vi "DVR Example.vi"() -> ()   [LabVIEW 2015]
uses:
  <vilib>/Erdos Miller/LV-VI/Check Out Ref.vi
  <vilib>/Erdos Miller/LV-VI/Check In Ref.vi
  <vilib>/Erdos Miller/LV-Async/async-xnode/LV-Async.xnode
  <vilib>/Erdos Miller/LV-Async/await-xnode/LV-Await.xnode
  <vilib>/Erdos Miller/LV-VI/LV-VI.lvlib
panel:
  out "data value out 2":dbl
  out "error out 2":errorcluster
  out "error out":errorcluster
  out "data value out":dbl
  in  "data value":dbl
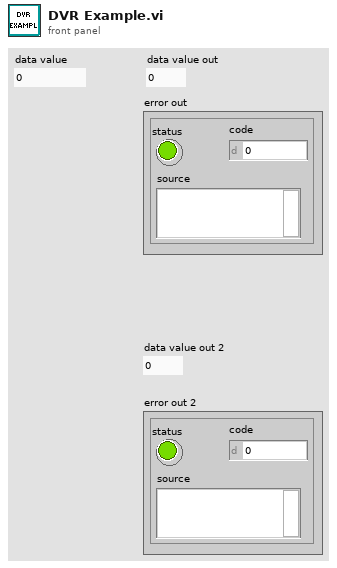
[diagram p1: front panel]
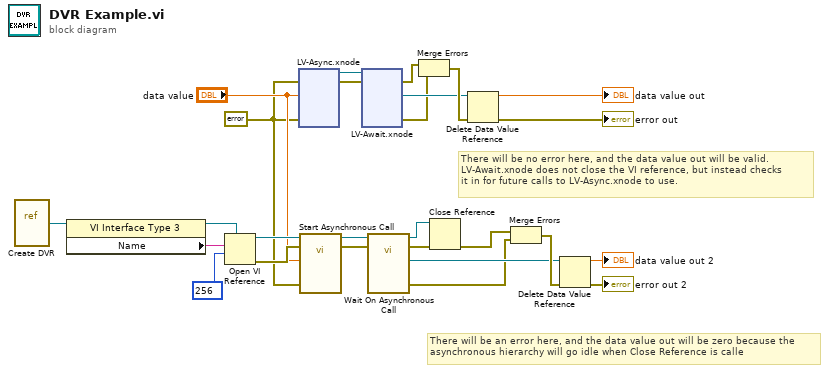
[diagram p0: block diagram]
diagram:
  w1 = errorcluster {"status"=FALSE, "code"=0, "source"=""} ("error in (no error)")
  # "There will be no error here, and the data value out will be valid.\nLV-Await.xnode does not close the VI reference, but instead checks\nit in for future calls to LV-Async.xnode to use."
  # "There will be an error here, and the data value out will be zero because the\nasynchronous hierarchy will go idle when Close Reference is calle"
  n1 = vi-ref "Create DVR.vi"() -> (w25:refnum<vi>)
  n2 = property class="VI Interface Type 3"(reference=w25) -> (reference out=w23:refnum<vi>, "Name"=w24:string)  [unwired: 1 in, 1 out]
  n3 = Open VI Reference(type specifier VI Refnum (for type only)=w23, vi path=w24, options=256) -> (vi reference=w21:refnum<vi>, error out=w20:errorcluster)  [unwired: 3 in]
  n4 = xnode "LV-Async.xnode"("Error In"=w1, "error in (no error)"=w1, "data value"="data value") -> ("Error Out"=w7:errorcluster, "VI Ref"=w6:refnum<vi>)
  n5 = call-by-ref "Start Asynchronous Call"(reference=w21, error in=w20, 8:"error in (no error)"=w1, "data value"="data value") -> (reference out=w8:refnum<vi>, error out=w19:errorcluster)  [unwired: 8 in, 2 out]
  n6 = xnode "LV-Await.xnode"("Error In"=w7, "VI Ref"=w6) -> ("Error Out"=w3:errorcluster, "error out"=w4:errorcluster, "data value reference"=w5:refnum<data-value>)
  n7 = call-by-ref "Wait On Asynchronous Call"(reference=w8, error in=w19) -> (reference out=w17:refnum<vi>, error out=w18:errorcluster, 0:"error out"=w9:errorcluster, "data value reference"=w11:refnum<data-value>)  [unwired: 10 in]
  n8 = Merge Errors(w3, w4) -> (w16:errorcluster)
  n9 = Close Reference(reference=w17, error in (no error)=w18) -> (error out=w10:errorcluster)
  n10 = Delete Data Value Reference(data value reference=w5, error in=w16) -> (data value=→"data value out":dbl, error out=→"error out":errorcluster)
  n11 = Merge Errors(w10, w9) -> (w13:errorcluster)
  n12 = Delete Data Value Reference(data value reference=w11, error in=w13) -> (data value=→"data value out 2":dbl, error out=→"error out 2":errorcluster)
